vi "Read IODevInfo.vi"(8 "error in (no error)":errorcluster, 11 "IO Device in":refnum<class "IO Device.lvclass">) -> (0 "error out":errorcluster, 2 "IODevInfo.lvclass":refnum<class "IODevInfo.lvclass">, 3 "IO Device out":refnum<class "IO Device.lvclass">)   [LabVIEW 2015, in "IO Device.lvlib" / "IO Device.lvclass"]
uses:
  IO Device.lvclass
  IODevInfo.lvclass
  IO Device.lvclass/IO Device.ctl
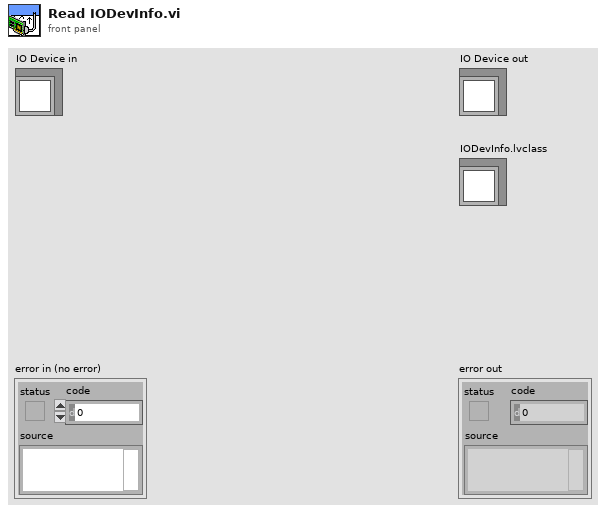
[diagram p1: front panel]
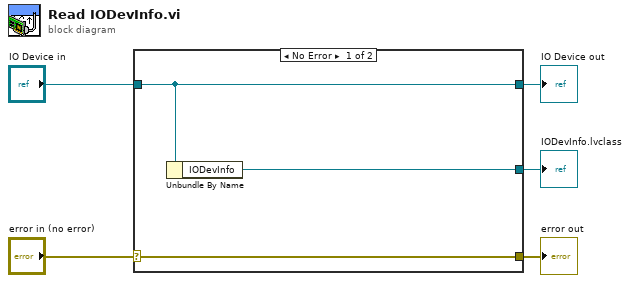
[diagram p0: block diagram]
diagram:
  n1 = case shown="No Error" "error in (no error)" {
    selector: "error in (no error)" -> [w8 w9]
    tunnel: [w8 w9] -> w4
    tunnel: [w7 w10] -> w2
    tunnel: "IO Device in" -> [w7 w10]
    tunnel: [w6 _] -> w1
    frame No Error {
      n2 = Unbundle By Name(w7) -> ("IODevInfo"=w6:refnum<class "IODevInfo.lvclass">)
    }
    frame Error {
    }
  }
  "error out" <- w4
  "IO Device out" <- w2
  "IODevInfo.lvclass" <- w1
